vi "Main.vi"() -> ()   [LabVIEW 2021, in "Instrument Studio Plug-In Template.lvlib"]
doc: "This template is for the Queued Message Handler design pattern.\n\nThe Event Handling Loop generates messages based on user interface actions.\n\nThe Message Handling Loop processes messages generated by the Event Handling Loop, or by other messages. The messages are string values, so new messages can be added easily to the Message Cases case structure in the Message Handling Loop. Each message cluster can also provide an optional value for Message Data, which is a variant that can be converted to whatever message-specific data is required."
uses:
  Instrument Studio Plug-In Template.lvlib
  <vilib>/Plug-In SDKs/InstrumentStudio SDK/InstrumentStudioPluginSDK.lvlibp/Plugin Events Enum.ctl
  controls/Configuration.ctl
  377644f2-3ba0-40c2-9637-345728516e3e.vi
  dd0e9e37-20d8-45cf-b11e-f419cd56f172.vi
  377644f2-3ba0-40c2-9637-345728516e3e.vi/6651a77e-856e-4bcd-af5a-c0c13b264cc1.vi
  dd0e9e37-20d8-45cf-b11e-f419cd56f172.vi/331b549c-fcf8-43d9-8a1e-5b3c0091a99c.vi
  subVIs/Message Queue/Enqueue Message (Single).vi
  <vilib>/JDP Science/JSONtext/JSON text to Variant.vi
  <vilib>/Utility/error.llb/Error Cluster From Error Code.vi
  <vilib>/JDP Science/JSONtext/Variant to JSON Text.vi
  <vilib>/JDP Science/JSONtext/LVClass Serializer/JSONtext LVClass Serializer.lvclass
  <vilib>/ErrorRing/Error Ring.xnode
  <vilib>/Plug-In SDKs/InstrumentStudio SDK/InstrumentStudioPluginSDK.lvlibp/Plugin Session.lvclass
  <vilib>/Plug-In SDKs/InstrumentStudio SDK/InstrumentStudioPluginSDK.lvlibp
panel:
  in  "Boolean In":bool
  in  "Numeric In":dbl
  in  "String In":string
  in  "Running":bool
  in  "Session Id":u64
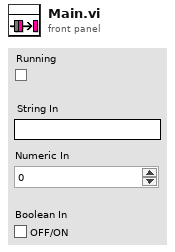
[diagram p1: front panel]
types:
  T1 = typedef "Instrument Studio Plug-In Template.lvlib/Configuration.ctl" = cluster{"String In":string, "Numeric In":dbl, "Boolean":bool}
  T2 = typedef "InstrumentStudioPluginSDK.lvlibp/Plugin Events Enum.ctl" = enum16{"Shutdown", "Project Saved", "Stop All Outputs"}
  T3 = typedef "InstrumentStudioPluginSDK.lvlibp/Event Registration Refnum.ctl" = refnum<event-registration>
  T4 = typedef "Instrument Studio Plug-In Template.lvlib/All Message Queues.ctl" = cluster{"UI":refnum<queue>}
  T5 = cluster{"Event Refnum":T3, "Event Registration Refnum":refnum<event-registration>}
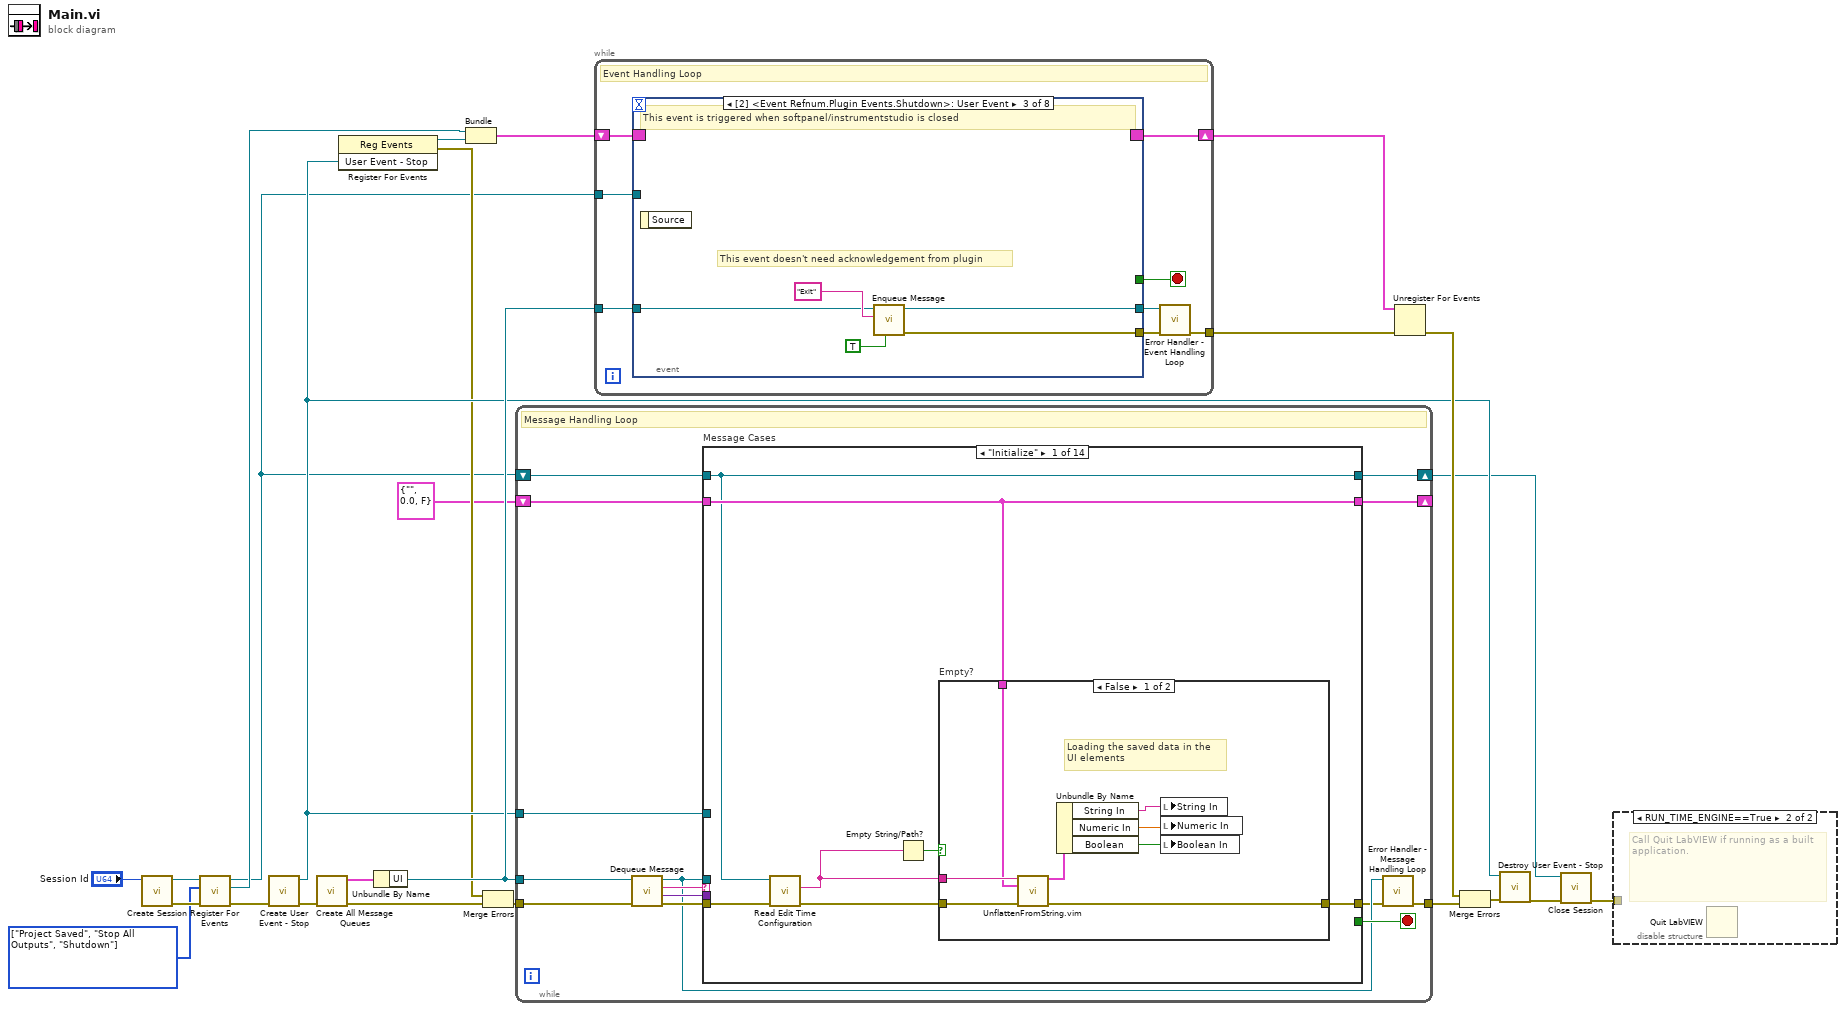
[diagram p0: block diagram]
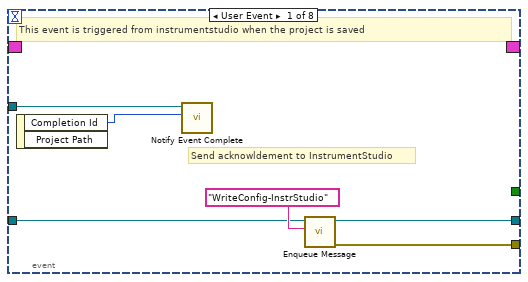
[diagram p3: hidden frame]
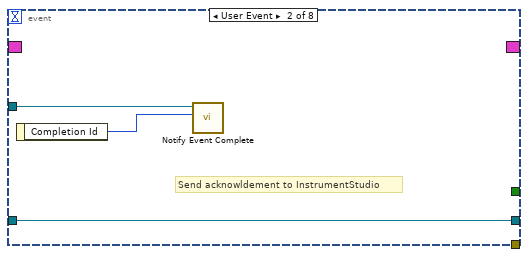
[diagram p4: hidden frame]
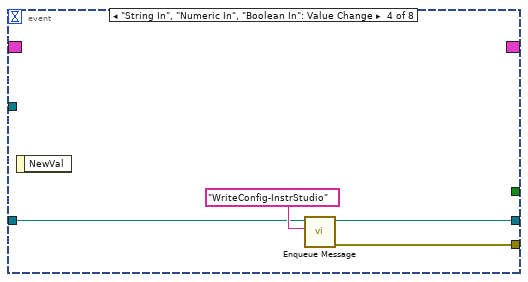
[diagram p5: hidden frame]
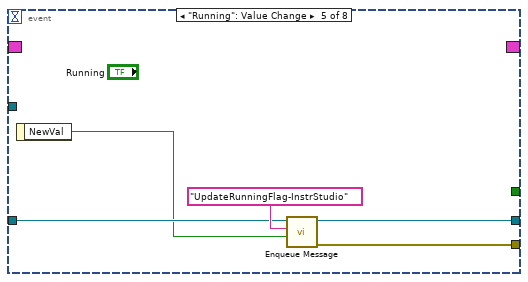
[diagram p6: hidden frame]
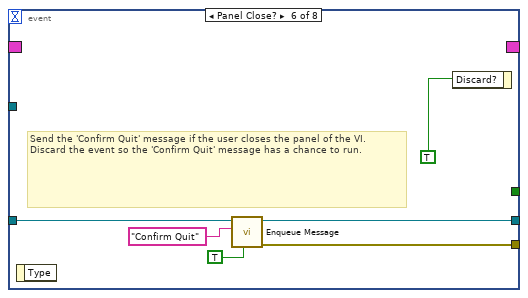
[diagram p7: hidden frame]
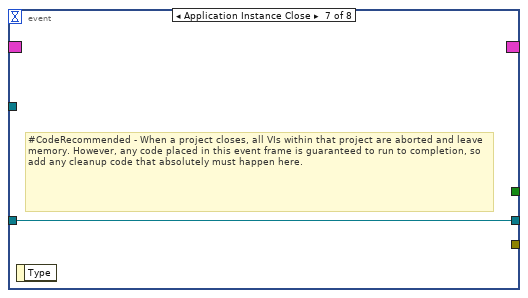
[diagram p8: hidden frame]
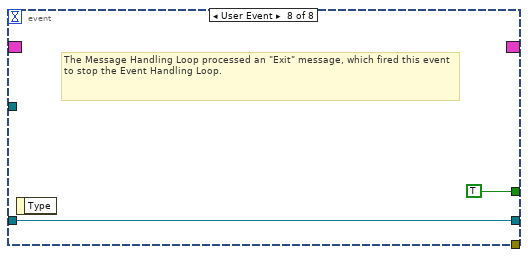
[diagram p9: hidden frame]
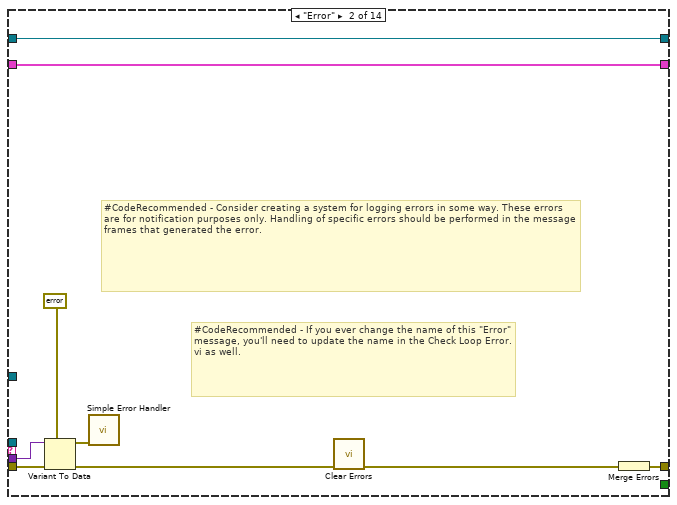
[diagram p11: hidden frame]
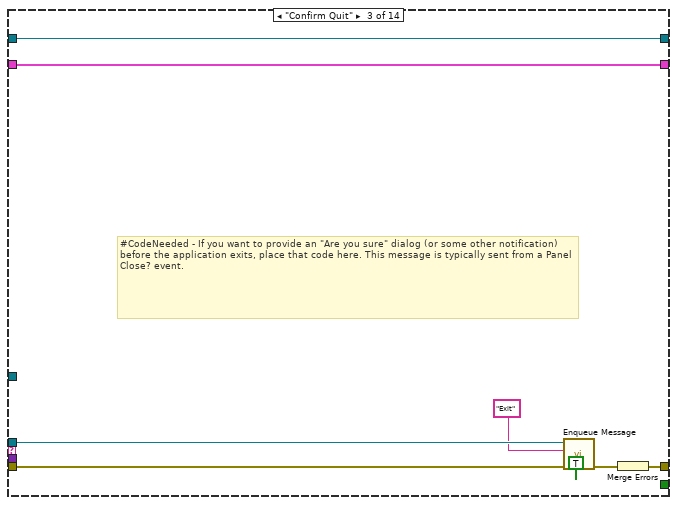
[diagram p12: hidden frame]
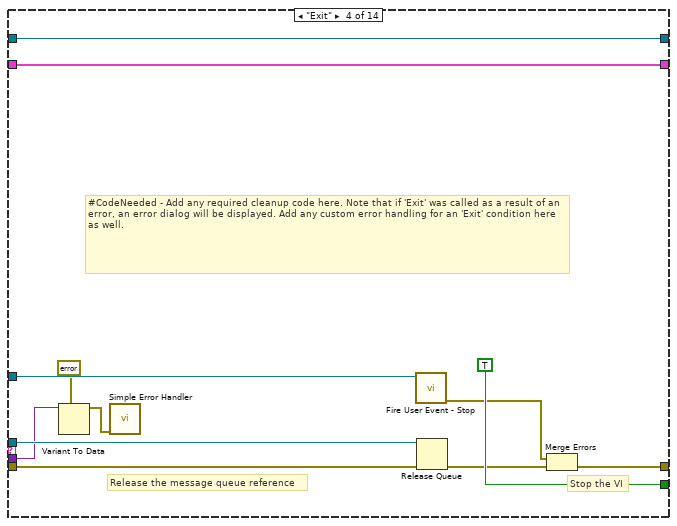
[diagram p13: hidden frame]
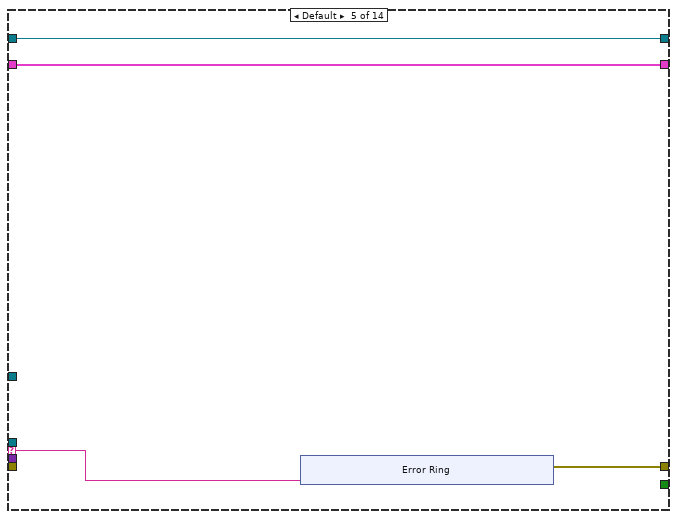
[diagram p14: hidden frame]
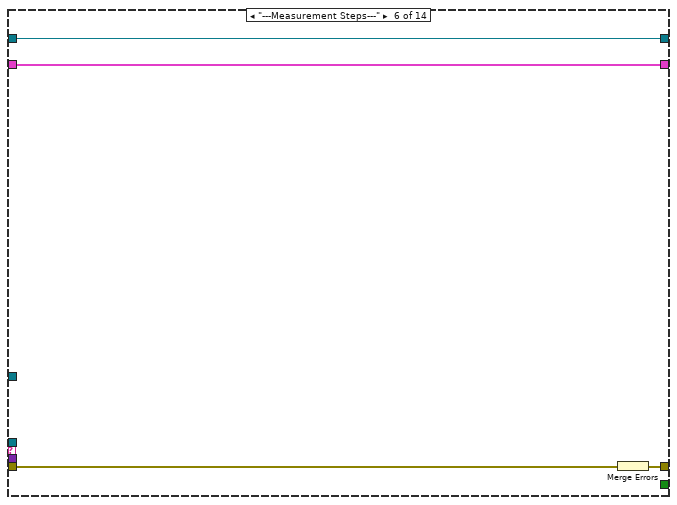
[diagram p15: hidden frame]
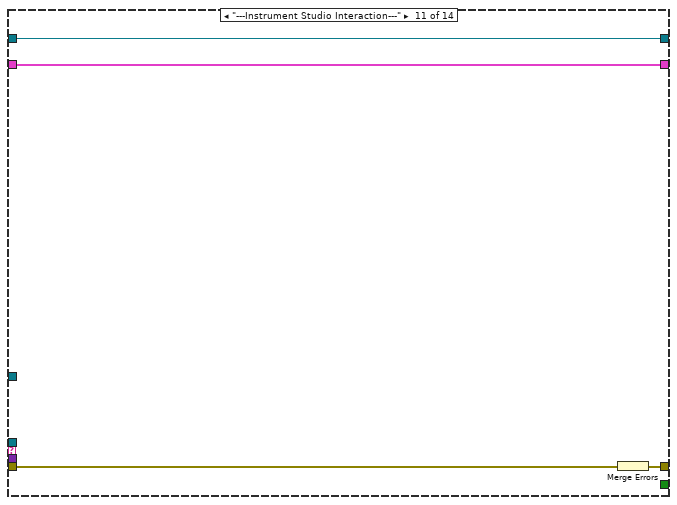
[diagram p20: hidden frame]
diagram:
  w9 = T2[] [enum."Project Saved", enum."Stop All Outputs", enum."Shutdown"] items=["Shutdown", "Project Saved", "Stop All Outputs"] ("Events To Register")
  n1 = call <vilib>:"Create Session.vi"("Session Id"="Session Id") -> ("error out"=w12:errorcluster, "Session out"=w10:refnum<class "Plugin Session.lvclass">)  [unwired: 6 in, 3 out]
  n2 = call <vilib>:"Register For Events.vi"("error in (no error)"=w12, "Events To Register"=w9, "Session in"=w10) -> ("error out"=w11:errorcluster, "Event Refnum"=w6:T3, "Session out"=w2:refnum<class "Plugin Session.lvclass">)  [unwired: 6 in]
  n3 = call "Create User Event - Stop.vi"("error in (no error)"=w11) -> ("error out"=w21:errorcluster, "User Event - Stop"=w16:refnum<user-event>)  [unwired: 9 in]
  n4 = call "Create All Message Queues.vi"("error in (no error)"=w21) -> ("error out"=w25:errorcluster, "Message Queues out"=w24:T4)  [unwired: 9 in]
  n5 = register-events(w16) -> (reference out=w8:refnum<event-registration>, error out=w14:errorcluster)  [unwired: 2 in]
  n6 = Unbundle By Name(w24) -> ("UI"=w22:refnum<queue>)
  n7 = Bundle("Event Refnum"=w6, "Event Registration Refnum"=w8) -> (w7:T5)  [unwired: 1 in]
  n8 = Merge Errors(w14, w25) -> (w15:errorcluster)
  n9 = while {
    tunnel: w22 -> [w33]
    tunnel: w16 -> [w38]
    tunnel: w15 -> [w37]
    tunnel: [w31] -> w23
    shift-right: [w28] -> w5
    shift-left: w2 -> [w29]
    shift-right: [w27] -> _
    shift-left: T1 {"String In"="", "Numeric In"=0.0, "Boolean"=FALSE} ("Configuration") -> [w26]
    stop <- w39 stop-if-true
    # "Message Handling Loop"
    n10 = call "Dequeue Message.vi"("error in (no error)"=w37, "Message Queue"=w33) -> ("error out"=w36:errorcluster, "Message Data"=w34:variant, "Message"=w35:string, "dup Message Queue"=w32:refnum<queue>)  [unwired: 6 in]
    n11 = case "Message Cases" shown="\"Initialize\"" w35 {
      selector: w35 -> [_ _ _ _ w87 _ _ _ _ _ _ _ _ _]
      tunnel: w32 -> [_ _ w69 w84 _ _ _ _ _ _ _ _ _ _]
      tunnel: w36 -> [w40 w64 w72 w78 _ w99 w102 w105 w108 w111 w115 w121 w128 w132]
      tunnel: [w45 w59 w71 w81 w88 w98 w102 w105 w108 w111 w114 w122 w126 w138] -> w30
      tunnel: [_ _ _ TRUE _ _ _ _ _ _ _ _ _ _] -> w39
      tunnel: w34 -> [_ w63 _ w75 _ _ _ _ _ _ _ w120 _ _]
      tunnel: w38 -> [_ _ _ w80 _ _ _ _ _ _ _ _ _ _]
      tunnel: w29 -> [w43 w58 w66 w74 w86 w97 w101 w104 w107 w110 w113 w124 w129 w140]
      tunnel: [w43 w58 w66 w74 w86 w97 w101 w104 w107 w110 w113 w123 w127 w139] -> w28
      tunnel: [w46 w57 w65 w73 w85 w96 w100 w103 w106 w109 w112 w116 w125 w133] -> w27
      tunnel: w26 -> [w46 w57 w65 w73 w85 w96 w100 w103 w106 w109 w112 w116 w125 w137]
      frame "Initialize" {
        # "Initialize - All initialization work should take place in this message, since other loops can potentially enqueue messages that execute immediately after this one."
        n12 = call <vilib>:"Read Edit Time Configuration.vi"("error in (no error)"=w40, "Session in"=w43) -> ("error out"=w41:errorcluster, "Edit Time Configuration"=w42:string)  [unwired: 7 in, 1 out]
        n13 = Empty String/Path?(string/path=w42) -> (empty?=w44:bool)
        n14 = case "Empty?" shown="False" w44 {
          tunnel: w46 -> [w50 _]
          tunnel: [w48 w55] -> w45
          tunnel: w41 -> [w47 w55]
          tunnel: w42 -> [w51 _]
          frame False {
            # "Loading the saved data in the \nUI elements"
            n15 = call "UnflattenFromString.vim"("Flattened Data"=w51, "Data Type"=w50, "error in"=w47) -> ("Data Out"=w49:T1, "error out"=w48:errorcluster)  [unwired: 11 in]
            n16 = Unbundle By Name(w49) -> ("String In"=w54:string, "Numeric In"=w53:dbl, "Boolean"=w52:bool)
            n17 = local write "String In"(w54) -> ()
            n18 = local write "Numeric In"(w53) -> ()
            n19 = local write "Boolean In"(w52) -> ()
          }
          frame True {
          }
        }
      }
      frame "Error" {
        # "#CodeRecommended - If you ever change the name of this \"Error\" message, you'll need to update the name in the Check Loop Error.vi as well."
        # "#CodeRecommended - Consider creating a system for logging errors in some way. These errors are for notification purposes only. Handling of specific errors should be performed in the message frames that generated the error."
        # "Error - Display an error dialog. This message is sent by the \"Error Handler\" VIs at the end of other loops in this application."
        n20 = Variant To Data(error in=w64, type=errorcluster {"status"=FALSE, "code"=0, "source"=""} ("error constant"), Variant=w63) -> (data=w61:errorcluster, error out=w60:errorcluster)
        n21 = call <vilib>:"Simple Error Handler.vi"("error in (no error)"=w61) -> ()  [unwired: 4 in, 5 out]
        n22 = call <vilib>:"Clear Errors.vi"("error in (no error)"=w60) -> ("error out"=w56:errorcluster)  [unwired: 5 in, 1 out]
        n23 = Merge Errors(w56) -> (w59:errorcluster)
      }
      frame "Confirm Quit" {
        # "#CodeNeeded - If you want to provide an \"Are you sure\" dialog (or some other notification) before the application exits, place that code here. This message is typically sent from a Panel Close? event."
        # "Confirm Quit - Message that can confirm whether or not the user wants to exit the application."
        n24 = call-poly "Enqueue Message.vi"("Priority Message? (F)"=TRUE, "error in (no error)"=w72, "Message"="Exit", "Message Queue"=w69) -> ("error out"=w70:errorcluster)  [unwired: 6 in, 1 out]
        n25 = Merge Errors(w70) -> (w71:errorcluster)
      }
      frame "Exit" {
        # "Stop the VI"
        # "Release the message queue reference"
        # "#CodeNeeded - Add any required cleanup code here. Note that if 'Exit' was called as a result of an error, an error dialog will be displayed. Add any custom error handling for an 'Exit' condition here as well."
        # "Exit - Exit the application."
        n26 = Variant To Data(type=errorcluster {"status"=FALSE, "code"=0, "source"=""} ("error constant"), Variant=w75) -> (data=w76:errorcluster)  [unwired: 1 in, 1 out]
        n27 = call <vilib>:"Simple Error Handler.vi"("error in (no error)"=w76) -> ()  [unwired: 4 in, 5 out]
        n28 = call "Fire User Event - Stop.vi"("User Event - Stop"=w80) -> ("error out"=w79:errorcluster)  [unwired: 10 in]
        n29 = Release Queue(queue=w84, error in (no error)=w78) -> (error out=w82:errorcluster)  [unwired: 1 in, 2 out]
        n30 = Merge Errors(w79, w82) -> (w81:errorcluster)
      }
      frame Default {
        # "'Default' case only runs if there is a message that isn't defined in any of the other cases.  Output a programming error."
        n31 = xnode "Error Ring"("parameter 0"=w87) -> ("error out"=w88:errorcluster)
      }
      frame "---Measurement Steps---" {
        # "Duplicate this frame when creating new messages.  Change this comment in the duplicated frame to describe this message."
        n32 = Merge Errors(w99) -> (w98:errorcluster)
      }
      frame "InstrumentSetup" {
      }
      frame "DUTControl" {
      }
      frame "Measurement" {
      }
      frame "Analysis" {
      }
      frame "---Instrument Studio Interaction---" {
        # "Duplicate this frame when creating new messages.  Change this comment in the duplicated frame to describe this message."
        n33 = Merge Errors(w115) -> (w114:errorcluster)
      }
      frame "UpdateRunningFlag-InstrStudio" {
        # "Updates the running flag in \nInstrumentStudio"
        n34 = Variant To Data(error in=w121, type=TRUE, Variant=w120) -> (data=w118:bool, error out=w117:errorcluster)
        n35 = call <vilib>:"Update Running State.vi"("error in (no error)"=w117, "Is Running"=w118, "Plugin Session in"=w124) -> ("error out"=w122:errorcluster, "Plugin Session out"=w123:refnum<class "Plugin Session.lvclass">)  [unwired: 7 in]
      }
      frame "ReadISProjectPath" {
        # "Reads the InstrumentStudio project path"
        n36 = call <vilib>:"Read Project Path.vi"("error in (no error)"=w128, "Session in"=w129) -> ("error out"=w126:errorcluster, "Session out"=w127:refnum<class "Plugin Session.lvclass">)  [unwired: 7 in, 1 out]
      }
      frame "WriteConfig-InstrStudio" {
        # "Saving the control inputs\nin the instrumentStudio object"
        n37 = Bundle By Name(cluster=w137, "String In"="String In", "Numeric In"="Numeric In", "Boolean"="Boolean In") -> (w133:T1)
        n38 = call "FlattenToString.vim"("Anything"=w133, "error in"=w132) -> ("Flattened Data"=w131:string, "error out"=w130:errorcluster)  [unwired: 12 in]
        n39 = call <vilib>:"Write Edit Time Configuration.vi"("error in (no error)"=w130, "Edit Time Configuration"=w131, "Session in"=w140) -> ("error out"=w138:errorcluster, "Session out"=w139:refnum<class "Plugin Session.lvclass">)  [unwired: 7 in]
      }
    }
    n40 = call "Error Handler - Message Handling Loop.vi"("error in (no error)"=w30, "Message Queue"=w32) -> ("dup error in"=w31:errorcluster)  [unwired: 8 in, 1 out]
  }
  n41 = while {
    tunnel: w22 -> [w148]
    shift-right: [w146] -> w18
    shift-left: w7 -> [w147]
    tunnel: [w142] -> w17
    tunnel: w2 -> [w141]
    stop <- w144 stop-if-true
    # "Event Handling Loop"
    n42 = event shown="[2] <Event Refnum.Plugin Events.Shutdown>: User Event" {
      selector: w147 -> [_ _ _ _ _ _ _ _]
      dyn-events: [_ _ _ _ _ _ _ _] -> w146
      timeout: _ -> [_ _ _ _ _ _ _ _]
      tunnel: [_ _ _ _ _ _ _ TRUE ("Discard?")] -> w144
      tunnel: w148 -> [w151 w157 w158 w165 w170 w176 w178 w180]
      tunnel: [w149 _ w159 w163 w168 w175 _ _] -> w145
      tunnel: [w150 w157 w160 w164 w169 w174 w178 w180] -> w143
      tunnel: w141 -> [w154 w156 _ _ _ _ _ _]
      event User Event {
        # "Send acknowldement to InstrumentStudio"
        # "This event is triggered from instrumentstudio when the project is saved"
        n43 = event-data() -> ("Completion Id"=w153:i64)  [unwired: 1 in, 1 out]
        n44 = call <vilib>:"Notify Event Complete.vi"("Completion Id"=w153, "Session in"=w154) -> ()  [unwired: 8 in, 2 out]
        n45 = call-poly "Enqueue Message.vi"("Message"="WriteConfig-InstrStudio", "Message Queue"=w151) -> ("error out"=w149:errorcluster, "dup Message Queue"=w150:refnum<queue>)  [unwired: 8 in]
      }
      event User Event {
        # "Send acknowldement to InstrumentStudio"
        n46 = event-data() -> ("Completion Id"=w155:i64)  [unwired: 1 in]
        n47 = call <vilib>:"Notify Event Complete.vi"("Completion Id"=w155, "Session in"=w156) -> ()  [unwired: 8 in, 2 out]
      }
      event User Event {
        # "This event doesn't need acknowledgement from plugin"
        # "This event is triggered when softpanel/instrumentstudio is closed"
        n48 = event-data() -> ()  [unwired: 1 in, 1 out]
        n49 = call-poly "Enqueue Message.vi"("Priority Message? (F)"=TRUE, "Message"="Exit", "Message Queue"=w158) -> ("error out"=w159:errorcluster, "dup Message Queue"=w160:refnum<queue>)  [unwired: 7 in]
      }
      event "String In", "Numeric In", "Boolean In": Value Change {
        n50 = event-data() -> ()  [unwired: 1 in, 1 out]
        n51 = call-poly "Enqueue Message.vi"("Message"="WriteConfig-InstrStudio", "Message Queue"=w165) -> ("error out"=w163:errorcluster, "dup Message Queue"=w164:refnum<queue>)  [unwired: 8 in]
      }
      event "Running": Value Change {
        n52 = event-data() -> ("NewVal"=w167:bool)  [unwired: 1 in]
        n53 = call-poly "Enqueue Message.vi"("Message Data"=w167, "Message"="UpdateRunningFlag-InstrStudio", "Message Queue"=w170) -> ("error out"=w168:errorcluster, "dup Message Queue"=w169:refnum<queue>)  [unwired: 7 in]
      }
      event Panel Close? {
        # "Send the 'Confirm Quit' message if the user closes the panel of the VI. Discard the event so the 'Confirm Quit' message has a chance to run."
        n54 = event-data() -> ()  [unwired: 1 in, 1 out]
        n55 = call-poly "Enqueue Message.vi"("Priority Message? (F)"=TRUE, "Message"="Confirm Quit", "Message Queue"=w176) -> ("error out"=w175:errorcluster, "dup Message Queue"=w174:refnum<queue>)  [unwired: 7 in]
        n56 = event-data("Discard?"=TRUE) -> ()  [unwired: 1 in, 1 out]
      }
      event Application Instance Close {
        # "#CodeRecommended - When a project closes, all VIs within that project are aborted and leave memory. However, any code placed in this event frame is guaranteed to run to completion, so add any cleanup code that absolutely must happen here."
        n57 = event-data() -> ()  [unwired: 1 in, 1 out]
      }
      event User Event {
        # "The Message Handling Loop processed an \"Exit\" message, which fired this event to stop the Event Handling Loop."
        n58 = event-data() -> ()  [unwired: 1 in, 1 out]
      }
    }
    n59 = call "Error Handler - Event Handling Loop.vi"("error in (no error)"=w145, "Message Queue"=w143) -> ("dup error in"=w142:errorcluster)  [unwired: 8 in, 1 out]
  }
  n60 = Unregister For Events(event registration refnum=w18, error in=w17) -> (error out=w19:errorcluster)
  n61 = Merge Errors(w19, w23) -> (w20:errorcluster)
  n62 = call "Destroy User Event - Stop.vi"("error in (no error)"=w20, "User Event - Stop"=w16) -> ("error out"=w4:errorcluster)  [unwired: 9 in]
  n63 = call <vilib>:"Close Session.vi"("error in (no error)"=w4, "Session in"=w5) -> ("error out"=w3:errorcluster)  [unwired: 9 in]
  n64 = disable-structure shown="RUN_TIME_ENGINE==True" {
    disable-tunnel: w3 -> [_ _]
    frame condition #0 (active) {
    }
    frame condition #1 {
      # "Call Quit LabVIEW if running as a built application."
      n65 = Quit LabVIEW() -> ()  [unwired: 1 in]
    }
  }
